vi "Test AO Configuration.vi"(8 "error in (no error)":errorcluster, 11 "Instrument.Lockin in":refnum<class "Instrument.Lockin.lvclass">) -> (0 "error out":errorcluster, 3 "Instrument.Lockin out":refnum<class "Instrument.Lockin.lvclass">)   [LabVIEW 2019]
uses:
  src/Instrument.Lockin/Instrument.Lockin.lvclass
  src/Instrument.DAQ/Typedefs/AO.Channel--Cluster--Array.ctl
  src/Instrument.DAQ/Typedefs/AO.Channel--Cluster.ctl
  src/Instrument.DAQ/Typedefs/AO.Channel.Function--Enum.ctl
  <vilib>/addons/_JKI Toolkits/Caraya/classes/Assert/Assert Not Error.vi
  <userlib>/_OpenG.lib/numeric/numeric.llb/Random Number Within Range - I32__ogtk.vi
  <userlib>/_OpenG.lib/numeric/numeric.llb/Random Number Within Range - DBL__ogtk.vi
  <vilib>/addons/_JKI Toolkits/Caraya/classes/Assert/Assert Almost Equal_Float.vi
  <vilib>/addons/_JKI Toolkits/Caraya/classes/Assert/Assert Equal Value_Variant.vi
  <vilib>/addons/_JKI Toolkits/Caraya/classes/Test/Test.lvclass
  <vilib>/addons/_JKI Toolkits/Caraya/classes/Assert/Assert.lvclass
  src/Instrument.DAQ/Instrument.DAQ.lvclass
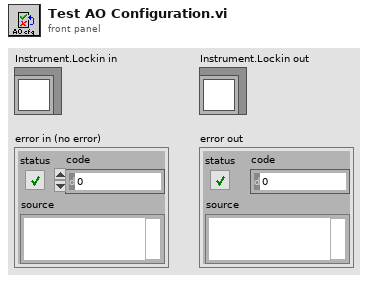
[diagram p1: front panel]
types:
  T1 = typedef "Instrument.Lockin.lvlib/Instrument.DAQ.lvclass/AO.Channel--Cluster--Array.ctl" = T2[]
  T2 = typedef "Instrument.Lockin.lvlib/Instrument.DAQ.lvclass/AO.Channel--Cluster.ctl" = cluster{"Enable?":bool, "Channel":i32, "Amplitude":dbl, "Offset":dbl, "Frequency":dbl, "Phase":dbl, "Function":T3, "Sweeping?":bool, "Limit AC":bool, "Limit DC?":bool, "Duty Cycle":bool}
  T3 = typedef "Instrument.Lockin.lvlib/Instrument.DAQ.lvclass/AO.Channel.Function--Enum.ctl" = enum16{"sine", "square", "triangle", "saw"}
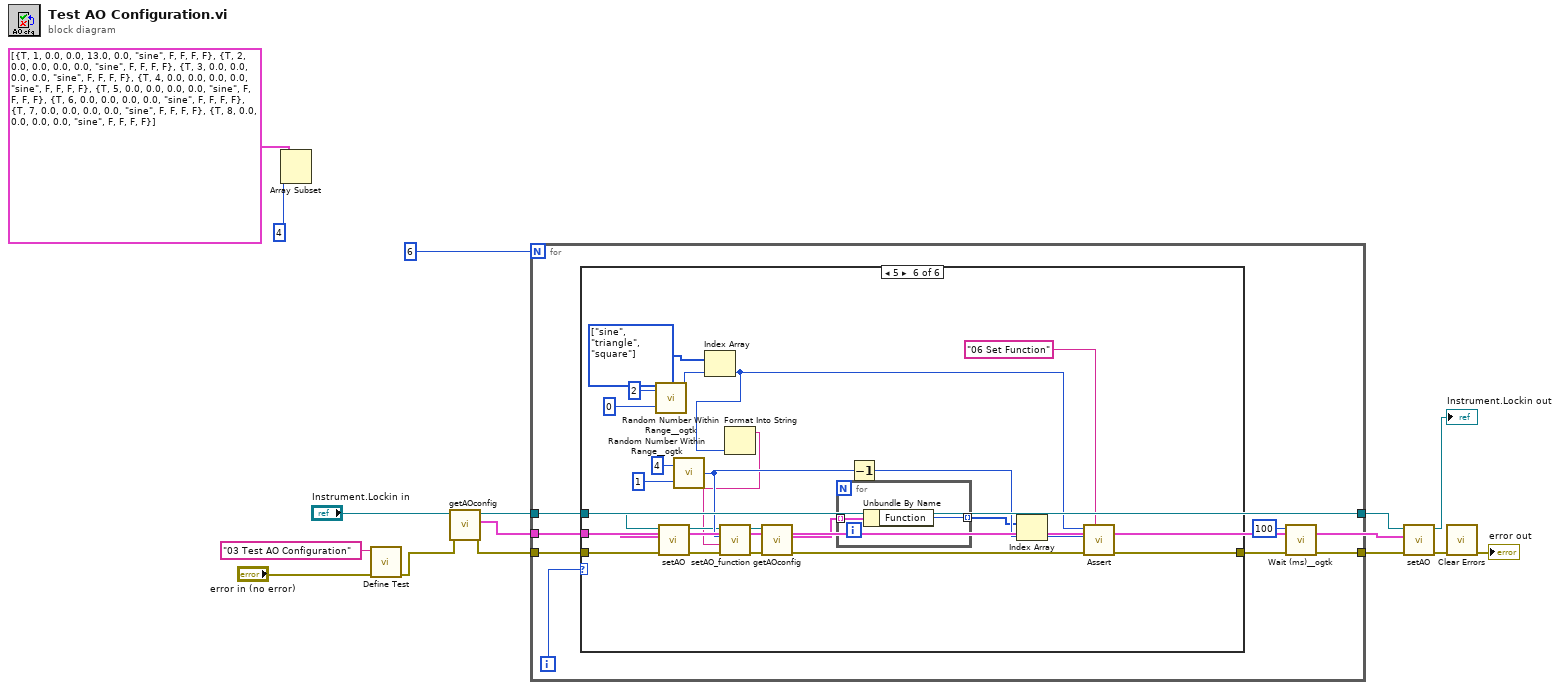
[diagram p0: block diagram]
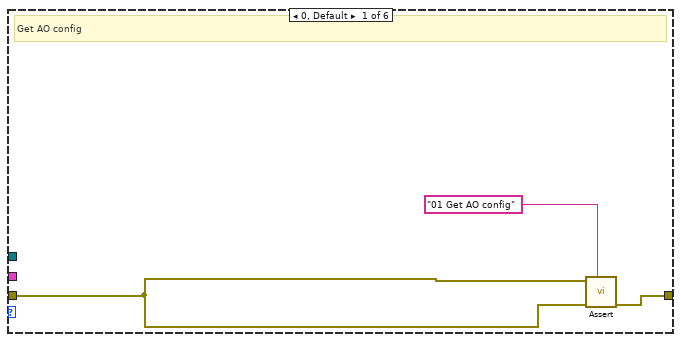
[diagram p2: hidden frame]
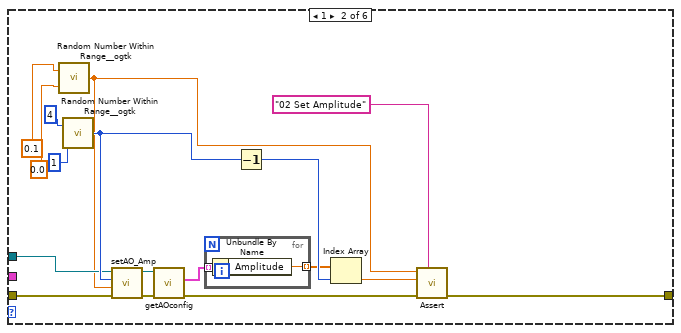
[diagram p3: hidden frame]
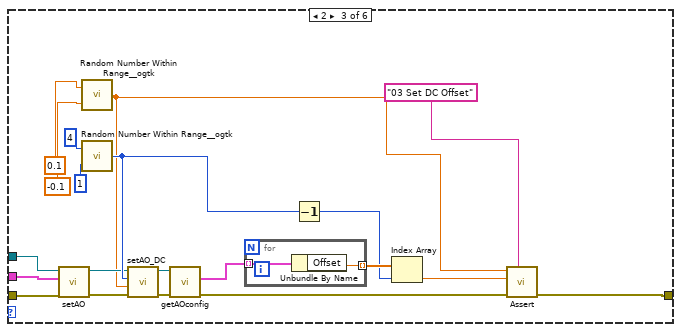
[diagram p4: hidden frame]
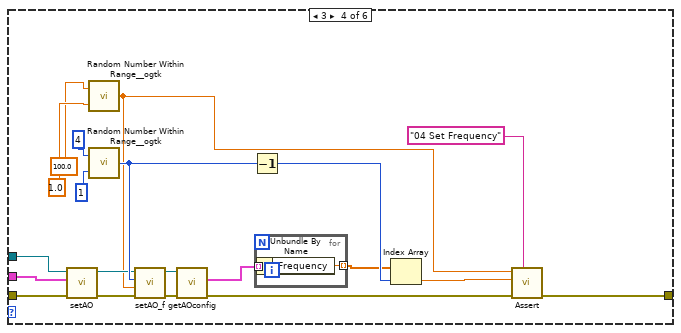
[diagram p5: hidden frame]
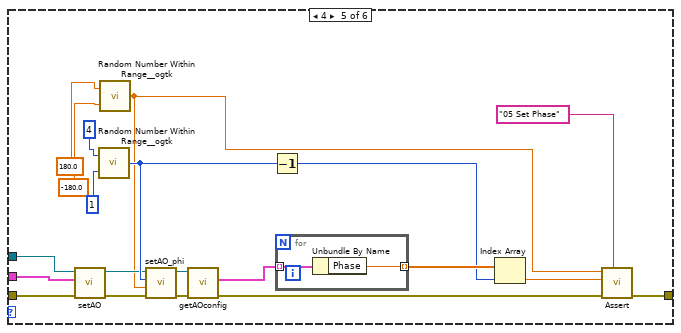
[diagram p6: hidden frame]
diagram:
  n1 = Array Subset(array=T1 [{"Enable?"=TRUE, "Channel"=1, "Amplitude"=0.0, "Offset"=0.0, "Frequency"=13.0, "Phase"=0.0, "Function"=enum."sine", "Sweeping?"=FALSE, "Limit AC"=FALSE, "Limit DC?"=FALSE, "Duty Cycle"=FALSE}, {"Enable?"=TRUE, "Channel"=2, "Amplitude"=0.0, "Offset"=0.0, "Frequency"=0.0, "Phase"=0.0, "Function"=enum."sine", "Sweeping?"=FALSE, "Limit AC"=FALSE, "Limit DC?"=FALSE, "Duty Cycle"=FALSE}, {"Enable?"=TRUE, "Channel"=3, "Amplitude"=0.0, "Offset"=0.0, "Frequency"=0.0, "Phase"=0.0, "Function"=enum."sine", "Sweeping?"=FALSE, "Limit AC"=FALSE, "Limit DC?"=FALSE, "Duty Cycle"=FALSE}, {"Enable?"=TRUE, "Channel"=4, "Amplitude"=0.0, "Offset"=0.0, "Frequency"=0.0, "Phase"=0.0, "Function"=enum."sine", "Sweeping?"=FALSE, "Limit AC"=FALSE, "Limit DC?"=FALSE, "Duty Cycle"=FALSE}, {"Enable?"=TRUE, "Channel"=5, "Amplitude"=0.0, "Offset"=0.0, "Frequency"=0.0, "Phase"=0.0, "Function"=enum."sine", "Sweeping?"=FALSE, "Limit AC"=FALSE, "Limit DC?"=FALSE, "Duty Cycle"=FALSE}, {"Enable?"=TRUE, "Channel"=6, "Amplitude"=0.0, "Offset"=0.0, "Frequency"=0.0, "Phase"=0.0, "Function"=enum."sine", "Sweeping?"=FALSE, "Limit AC"=FALSE, "Limit DC?"=FALSE, "Duty Cycle"=FALSE}, {"Enable?"=TRUE, "Channel"=7, "Amplitude"=0.0, "Offset"=0.0, "Frequency"=0.0, "Phase"=0.0, "Function"=enum."sine", "Sweeping?"=FALSE, "Limit AC"=FALSE, "Limit DC?"=FALSE, "Duty Cycle"=FALSE}, {"Enable?"=TRUE, "Channel"=8, "Amplitude"=0.0, "Offset"=0.0, "Frequency"=0.0, "Phase"=0.0, "Function"=enum."sine", "Sweeping?"=FALSE, "Limit AC"=FALSE, "Limit DC?"=FALSE, "Duty Cycle"=FALSE}] ("Channels: AO"), length=4) -> ()  [unwired: 1 in, 1 out]
  n2 = call <vilib>:"Define Test.vi"("error in (no error)"="error in (no error)", "Label (VI Title)"="03 Test AO Configuration") -> ("error out"=w5:errorcluster)  [unwired: 8 in, 1 out]
  n3 = call-dynamic "getAOconfig.vi"("error in (no error)"=w5, "Instrument.Lockin in"="Instrument.Lockin in") -> ("error out"=w4:errorcluster, "AOconfig"=w1:T1, "Instrument.Lockin out"=w3:refnum<class "Instrument.Lockin.lvclass">)  [unwired: 7 in]
  n4 = for {
    N: 6 -> [_]
    tunnel: w3 -> [w16]
    tunnel: w1 -> [w20]
    tunnel: w4 -> [w21]
    tunnel: [w18] -> w12
    tunnel: [w16] -> w2
    i -> [w22]
    n5 = case shown="5" w22 {
      tunnel: w16 -> [_ w32 w51 w73 w95 w120]
      tunnel: w21 -> [w23 w33 w52 w74 w94 w119]
      tunnel: w20 -> [_ _ w50 w67 w96 w121]
      tunnel: [w24 w28 w47 w69 w89 w115] -> w19
      frame 0, Default {
        # "Get AO config"
        n6 = call-poly <vilib>:"Assert.vi"("Label"="01 Get AO config", "error in (no error)"=w23, "Not Error?"=w23) -> ("error out"=w24:errorcluster)  [unwired: 7 in, 1 out]
      }
      frame 1 {
        n7 = call-poly <userlib>:"Random Number Within Range__ogtk.vi"("High"=0.1, "Low"=0.0) -> ("Random Number"=w31:dbl)  [unwired: 3 in]
        n8 = call-poly <userlib>:"Random Number Within Range__ogtk.vi"("High"=4, "Low"=1) -> ("Random Number"=w40:i32)  [unwired: 3 in]
        n9 = call-dynamic "setAO_Amp.vi"("error in (no error)"=w33, "Amplitude (V)"=w31, "AO Channel"=w40, "Instrument.Lockin in"=w32) -> ("error out"=w34:errorcluster, "Instrument.Lockin out"=w35:refnum<class "Instrument.Lockin.lvclass">)  [unwired: 6 in]
        n10 = call-dynamic "getAOconfig.vi"("error in (no error)"=w34, "Instrument.Lockin in"=w35) -> ("error out"=w29:errorcluster, "AOconfig"=w36:T1)  [unwired: 7 in, 1 out]
        n11 = for {
          tunnel: [w44] -> w37 mode=indexing
          tunnel: w36 -> [w43] mode=indexing
          n12 = Unbundle By Name(w43) -> ("Amplitude"=w44:dbl)
        }
        n13 = Decrement(x=w40) -> (x-1=w38:i32)
        n14 = Index Array(array=w37, index=w38) -> (element=w30:dbl)
        n15 = call-poly <vilib>:"Assert.vi"("Label"="02 Set Amplitude", "error in (no error)"=w29, "Actual"=w30, "Expected"=w31) -> ("error out"=w28:errorcluster)  [unwired: 6 in, 1 out]
      }
      frame 2 {
        n16 = call-dynamic "setAO.vi"("error in (no error)"=w52, "Channels: AO"=w50, "Instrument.Lockin in"=w51) -> ("error out"=w60:errorcluster, "Instrument.Lockin out"=w59:refnum<class "Instrument.Lockin.lvclass">)  [unwired: 7 in]
        n17 = call-poly <userlib>:"Random Number Within Range__ogtk.vi"("High"=0.1, "Low"=-0.1) -> ("Random Number"=w45:dbl)  [unwired: 3 in]
        n18 = call-poly <userlib>:"Random Number Within Range__ogtk.vi"("High"=4, "Low"=1) -> ("Random Number"=w63:i32)  [unwired: 3 in]
        n19 = call-dynamic "setAO_DC.vi"("error in (no error)"=w60, "DC (V)"=w45, "AO Channel"=w63, "Instrument.Lockin in"=w59) -> ("error out"=w53:errorcluster, "Instrument.Lockin out"=w54:refnum<class "Instrument.Lockin.lvclass">)  [unwired: 6 in]
        n20 = call-dynamic "getAOconfig.vi"("error in (no error)"=w53, "Instrument.Lockin in"=w54) -> ("error out"=w46:errorcluster, "AOconfig"=w64:T1)  [unwired: 7 in, 1 out]
        n21 = for {
          tunnel: w64 -> [w66] mode=indexing
          tunnel: [w65] -> w62 mode=indexing
          n22 = Unbundle By Name(w66) -> ("Offset"=w65:dbl)
        }
        n23 = Decrement(x=w63) -> (x-1=w61:i32)
        n24 = Index Array(array=w62, index=w61) -> (element=w49:dbl)
        n25 = call-poly <vilib>:"Assert.vi"("Label"="03 Set DC Offset", "error in (no error)"=w46, "Actual"=w49, "Expected"=w45) -> ("error out"=w47:errorcluster)  [unwired: 6 in, 1 out]
      }
      frame 3 {
        n26 = call-dynamic "setAO.vi"("error in (no error)"=w74, "Channels: AO"=w67, "Instrument.Lockin in"=w73) -> ("error out"=w78:errorcluster, "Instrument.Lockin out"=w77:refnum<class "Instrument.Lockin.lvclass">)  [unwired: 7 in]
        n27 = call-poly <userlib>:"Random Number Within Range__ogtk.vi"("High"=100.0, "Low"=1.0) -> ("Random Number"=w71:dbl)  [unwired: 3 in]
        n28 = call-poly <userlib>:"Random Number Within Range__ogtk.vi"("High"=4, "Low"=1) -> ("Random Number"=w85:i32)  [unwired: 3 in]
        n29 = call-dynamic "setAO_f.vi"("error in (no error)"=w78, "Frequency (Hz)"=w71, "AO Channel"=w85, "Instrument.Lockin in"=w77) -> ("error out"=w75:errorcluster, "Instrument.Lockin out"=w76:refnum<class "Instrument.Lockin.lvclass">)  [unwired: 6 in]
        n30 = call-dynamic "getAOconfig.vi"("error in (no error)"=w75, "Instrument.Lockin in"=w76) -> ("error out"=w68:errorcluster, "AOconfig"=w86:T1)  [unwired: 7 in, 1 out]
        n31 = Decrement(x=w85) -> (x-1=w80:i32)
        n32 = for {
          tunnel: w86 -> [w88] mode=indexing
          tunnel: [w87] -> w79 mode=indexing
          n33 = Unbundle By Name(w88) -> ("Frequency"=w87:dbl)
        }
        n34 = Index Array(array=w79, index=w80) -> (element=w72:dbl)
        n35 = call-poly <vilib>:"Assert.vi"("Label"="04 Set Frequency", "error in (no error)"=w68, "Actual"=w72, "Expected"=w71) -> ("error out"=w69:errorcluster)  [unwired: 6 in, 1 out]
      }
      frame 4 {
        n36 = call-dynamic "setAO.vi"("error in (no error)"=w94, "Channels: AO"=w96, "Instrument.Lockin in"=w95) -> ("error out"=w108:errorcluster, "Instrument.Lockin out"=w99:refnum<class "Instrument.Lockin.lvclass">)  [unwired: 7 in]
        n37 = call-poly <userlib>:"Random Number Within Range__ogtk.vi"("High"=4, "Low"=1) -> ("Random Number"=w107:i32)  [unwired: 3 in]
        n38 = call-poly <userlib>:"Random Number Within Range__ogtk.vi"("High"=180.0, "Low"=-180.0) -> ("Random Number"=w92:dbl)  [unwired: 3 in]
        n39 = call-dynamic "setAO_phi.vi"("error in (no error)"=w108, "Phase (°)"=w92, "AO Channel"=w107, "Instrument.Lockin in"=w99) -> ("error out"=w97:errorcluster, "Instrument.Lockin out"=w98:refnum<class "Instrument.Lockin.lvclass">)  [unwired: 6 in]
        n40 = call-dynamic "getAOconfig.vi"("error in (no error)"=w97, "Instrument.Lockin in"=w98) -> ("error out"=w90:errorcluster, "AOconfig"=w106:T1)  [unwired: 7 in, 1 out]
        n41 = Decrement(x=w107) -> (x-1=w104:i32)
        n42 = for {
          tunnel: w106 -> [w110] mode=indexing
          tunnel: [w109] -> w105 mode=indexing
          n43 = Unbundle By Name(w110) -> ("Phase"=w109:dbl)
        }
        n44 = Index Array(array=w105, index=w104) -> (element=w91:dbl)
        n45 = call-poly <vilib>:"Assert.vi"("Label"="05 Set Phase", "error in (no error)"=w90, "Actual"=w91, "Expected"=w92) -> ("error out"=w89:errorcluster)  [unwired: 6 in, 1 out]
      }
      frame 5 {
        w114 = T3[] [enum."sine", enum."triangle", enum."square"] items=["sine", "square", "triangle", "saw"] ("Function")
        n46 = call-poly <userlib>:"Random Number Within Range__ogtk.vi"("High"=2, "Low"=0) -> ("Random Number"=w113:i32)  [unwired: 3 in]
        n47 = call-dynamic "setAO.vi"("error in (no error)"=w119, "Channels: AO"=w121, "Instrument.Lockin in"=w120) -> ("error out"=w125:errorcluster, "Instrument.Lockin out"=w124:refnum<class "Instrument.Lockin.lvclass">)  [unwired: 7 in]
        n48 = call-poly <userlib>:"Random Number Within Range__ogtk.vi"("High"=4, "Low"=1) -> ("Random Number"=w131:i32)  [unwired: 3 in]
        n49 = Index Array(array=w114, index=w113) -> (element=w112:T3)
        n50 = Format Into String(w112) -> (resulting string=w111:string)  [unwired: 3 in, 1 out]
        n51 = call-dynamic "setAO_function.vi"("error in (no error)"=w125, "function"=w111, "AO Channel"=w131, "Instrument.Lockin in"=w124) -> ("error out"=w122:errorcluster, "Instrument.Lockin out"=w123:refnum<class "Instrument.Lockin.lvclass">)  [unwired: 6 in]
        n52 = call-dynamic "getAOconfig.vi"("error in (no error)"=w122, "Instrument.Lockin in"=w123) -> ("error out"=w117:errorcluster, "AOconfig"=w130:T1)  [unwired: 7 in, 1 out]
        n53 = for {
          tunnel: w130 -> [w135] mode=indexing
          tunnel: [w134] -> w126 mode=indexing
          n54 = Unbundle By Name(w135) -> ("Function"=w134:T3)
        }
        n55 = Decrement(x=w131) -> (x-1=w127:i32)
        n56 = Index Array(array=w126, index=w127) -> (element=w118:T3)
        n57 = call-poly <vilib>:"Assert.vi"("Label"="06 Set Function", "error in (no error)"=w117, "Actual"=w118, "Expected"=w112) -> ("error out"=w115:errorcluster)  [unwired: 6 in, 1 out]
      }
    }
    n58 = call <userlib>:"Wait (ms)__ogtk.vi"("error in (no error)"=w19, "milliseconds to wait"=u32 100) -> ("error out"=w18:errorcluster)  [unwired: 8 in, 1 out]
  }
  n59 = call-dynamic "setAO.vi"("error in (no error)"=w12, "Channels: AO"=w1, "Instrument.Lockin in"=w2) -> ("error out"=w14:errorcluster, "Instrument.Lockin out"=→"Instrument.Lockin out":refnum<class "Instrument.Lockin.lvclass">)  [unwired: 7 in]
  n60 = call <vilib>:"Clear Errors.vi"("error in (no error)"=w14) -> ("error out"=→"error out":errorcluster)  [unwired: 5 in, 1 out]
